vi "Laser_COM_both.vi"() -> ()   [LabVIEW 2014]
uses:
  <vilib>/Instr/_visa.llb/Select Event Type.ctl
  <vilib>/Instr/_visa.llb/VISA Configure Serial Port (Instr).vi
panel:
  in  "Freq":dbl(slide) caption="freq" min=59.9 max=1000.0 step=0.1 scale=59.9..1000.0 scale format="%#.1f"
  out "f kHz":dbl caption="Темп. модуля" format="%#_g kHz"
  out "7":bool
  out "6":bool
  out "4":bool
  out "5":bool
  out "3":bool
  out "2":bool
  out "1":bool
  out "0":bool
  out "DB25 ML":bool
  out "RS232 ML":bool
  in  "Control ML":bool
  out "on/off? 5":bool
  in  "Laser":bool
  out "Laser EM":bool caption="Излучение включено!"
  out "on/off? 3":bool
  out "on/off? 2":bool
  in  "Send":bool
  in  "write buffer":string caption="Передать команду"
  out "COM_connect":bool
  in  "Connect":bool
  out "SN:":string
  out "ID:":string
  out "Guide  laser":bool
  out "module temp":dbl caption="Темп. модуля" format="%#_g °C"
  in  "Power":dbl(slide) caption="Мощность излучения, %" min=0.0 max=100.0 step=0.5 scale=0.0..100.0 scale format="%#.2g"
  in  "Laser pilot":bool caption="Лазер пилот"
  in  "COM":refnum<visa-resource-name>="COM1" caption="Laser COM-port"
  out "read buffer":string caption="ОТВЕТ:"
  out "error out":errorcluster
  in  "error in (no error)":errorcluster
  # "ID:\n\nSN:"
  # "DB-25"
  # "RS-232"
  # "Блок  управления основным лазером"
  # "Мощьность  излучения, %"
  # "DB-25"
  # "Частота следования импульсов, кГц"
  # "T модуля -"
  # "Пилот Лазер"
  # "Терминал"
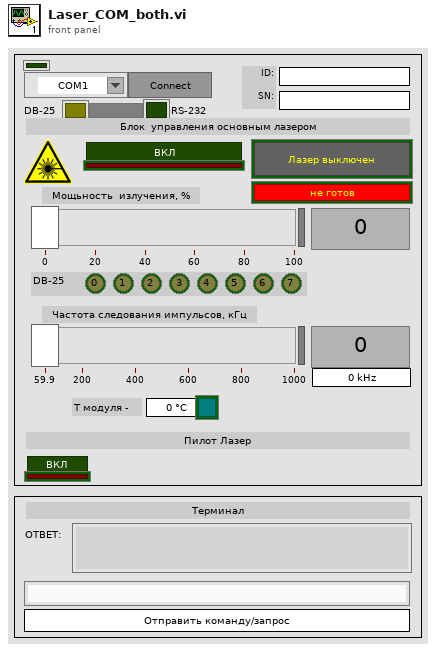
[diagram p1: front panel]
types:
  T1 = typedef "Select Event Type.ctl" = u32
  T2 = cluster{"Control by DB-25":bool, "Control by RS-232":bool, "AuxOFF control by DB-25":bool, "Guide laser control by DB-25":bool, "PRR controlled by Sync line ":bool, "Reserved[1]":bool, "The laser is in Sweep PRR mode":bool, "Modulation control by DB-25":bool, "The laser is in Jump PRR mode":bool, "Reserved[2]":bool, "Bitstream 1 (BS1) mode is active":bool, "Bitstream (BS) mode is active":bool}
  T3 = cluster{"Power control by DB-25":bool, "Reserved[1]":bool, "AuxOFF control by DB-25":bool, "Guide laser control by DB-25":bool, "Reserved[4]":bool, "Reserved[5]":bool, "Reserved[6]":bool, "Emission Modulation control by DB-25":bool, "The laser is in Jump PRR mode":bool, "Reserved[9]":bool, "Bitstream 1 (BS1) mode is active":bool, "Reserved[11]":bool, "PRR controlled by Sync line in DB-25":bool, "Emission Enable control by DB-25":bool, "APD mode is controlled by DB-25":bool, "Automatic latch":bool, "Reserved[16]":bool, "Reserved[17]":bool, "Reserved[18]":bool, "The laser is in Sweep PRR mode":bool, "The laser is in Follow PRR mode":bool, "Manual Prepump mode is active":bool, "Manual residual is controlled by DB-25":bool, "Reserved[23]":bool, "Reserved[24]":bool, "Guide laser safety function is not activated":bool, "Discharge circuit safety function is activated":bool, "Reserved[27]":bool, "Reserved[28]":bool, "Reserved[29]":bool, "Reserved[30]":bool, "Reserved[31]":bool}
  T4 = cluster{"Emergency stop":bool, "External syn frequency on pin 20 is above spec":bool, "External syn frequency on pin 20 is below spec":bool, "Laser ON time (pin 19 HIGH state) is lower spec":bool, "Laser ON time (pin 19 LOW state) is lower spec":bool, "Guide laser":bool, "Reserved [6]":bool, "Reserved [7]":bool, "Laser emission":bool, "Reserved [9]":bool, "Reserved [10]":bool, "Laser emission command was received by RS-232":bool, "Guide laser command was received by RS-232":bool, "24V Main supply voltage is in specified range":bool, "Laser uses 24V housekeeping supply":bool, "Laser uses 5V housekeeping supply":bool, "Manual Prepump is limited by it's max value 10000":bool}
  T5 = cluster{"Emergency stop":bool, "External PRR [1]":bool, "External PRR [2]":bool, "Reserved [3]":bool, "Reserved [4]":bool, "Guide laser":bool, "Reserved [6]":bool, "Reserved [7]":bool, "Laser emission":bool, "Reserved [9]":bool, "Reserved [10]":bool, "Laser emission command was received by RS-232":bool, "Guide laser command was received by RS-232":bool, "24V Main supply voltage is in specified range":bool, "HK supply voltage is in specified range":bool, "Emission Enable is switched by RS-232":bool, "Reserved [16]":bool, "Reserved [17]":bool, "Reserved [18]":bool, "Reserved [19]":bool, "Reserved [20]":bool, "Reserved [21]":bool, "Reserved [22]":bool, "Reserved [23]":bool, "Reserved [24]":bool, "Reserved [25]":bool, "Reserved [26]":bool, "Reserved [27]":bool, "Reserved [28]":bool, "Reserved [29]":bool, "Reserved [30]":bool, "Reserved [31]":bool}
  T6 = cluster{"D0 latched power setting":bool, "D1 latched power setting":bool, "D2 latched power setting":bool, "D3 latched power setting":bool, "D4 latched power setting":bool, "D5 latched power setting":bool, "D6 latched power setting":bool, "D7 latched power setting":bool, "D0 power setting":bool, "D1 power setting":bool, "D2 power setting":bool, "D3 power setting":bool, "D4 power setting":bool, "D5 power setting":bool, "D6 power setting":bool, "D7 power setting":bool, "Latch":bool, "23 AuxOFF Auxiliary Emission OFF":bool, "19 EM Emission Modulation":bool, "22 RG Guide laser control":bool, "20 Sync External Synchronization Input":bool, "18 EE Emission enable":bool, "10 Serial Input":bool, "13 Serial Clock":bool, "16 Laser status":bool, "21 Laser status":bool, "11 Laser status":bool, "12 Serial Output":bool, "24 Serial Enable":bool, "Reserved [29]":bool, "Reserved [30]":bool, "Reserved [31]":bool}
  T7 = cluster{"Module temp is out range":bool, "5V supply voltage is out range":bool, "High rack reflection":bool, "Reserved [1]":bool, "Normal Laser's status":bool, "Laser isn't ready to emmision":bool, "System error":bool, "Reserved [2]":bool}
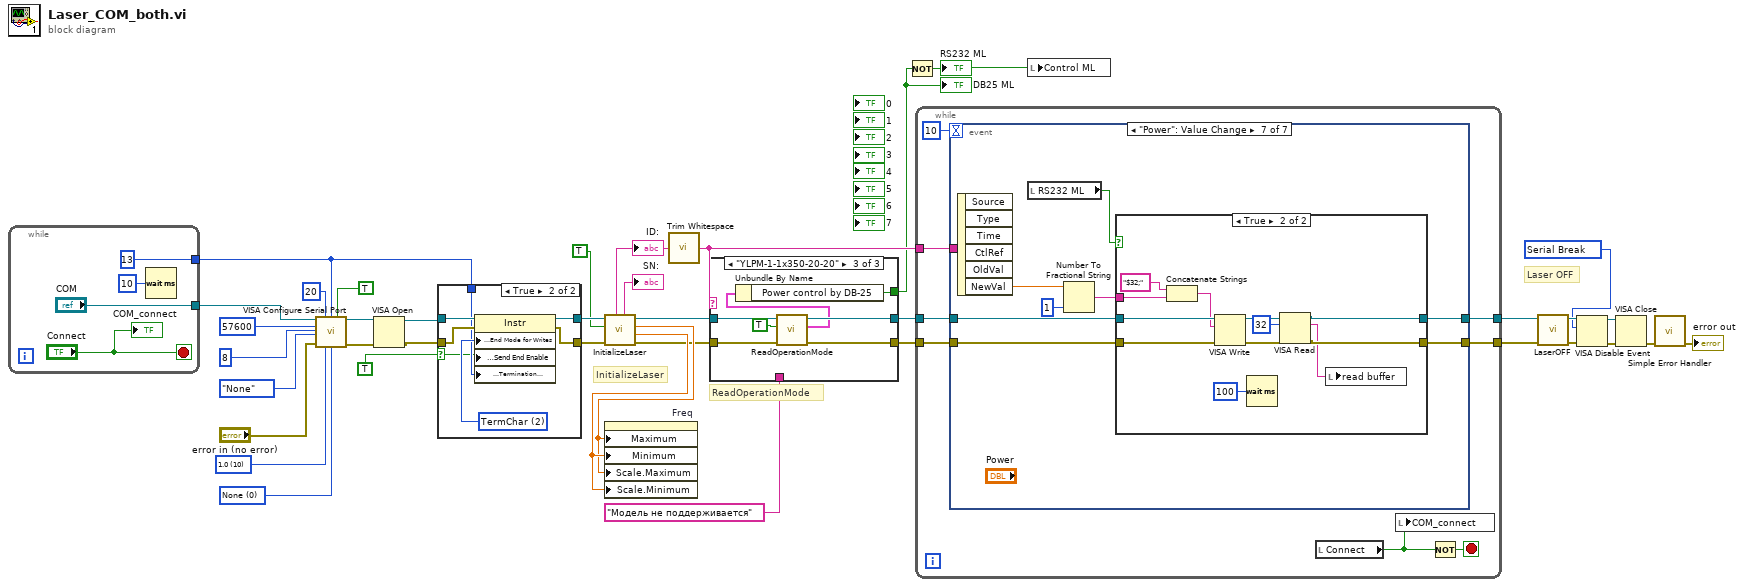
[diagram p0: block diagram]
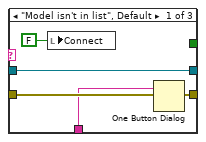
[diagram p2: hidden frame]
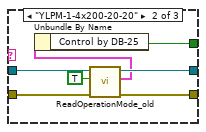
[diagram p3: hidden frame]
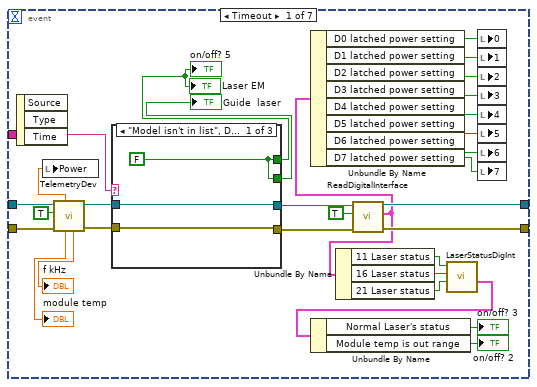
[diagram p4: hidden frame]
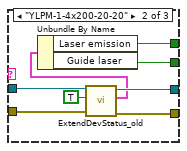
[diagram p5: hidden frame]
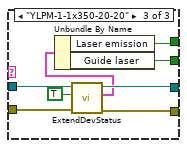
[diagram p6: hidden frame]
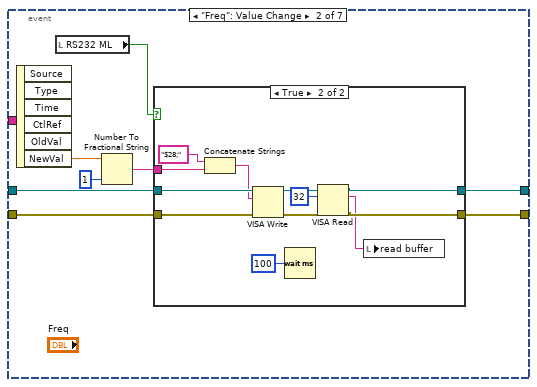
[diagram p7: hidden frame]
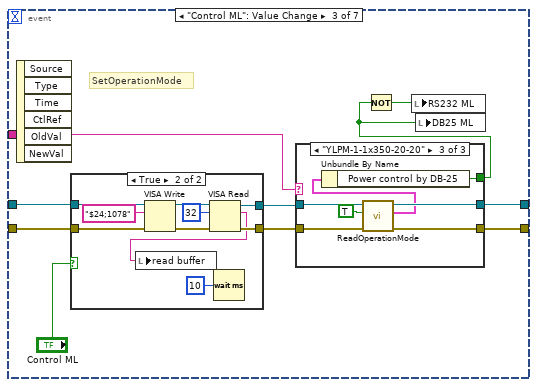
[diagram p9: hidden frame]
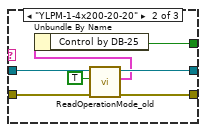
[diagram p11: hidden frame]
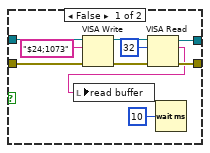
[diagram p12: hidden frame]
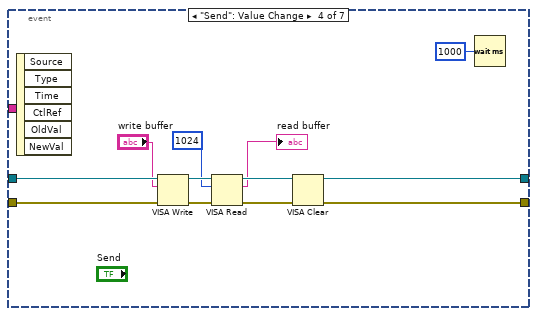
[diagram p13: hidden frame]
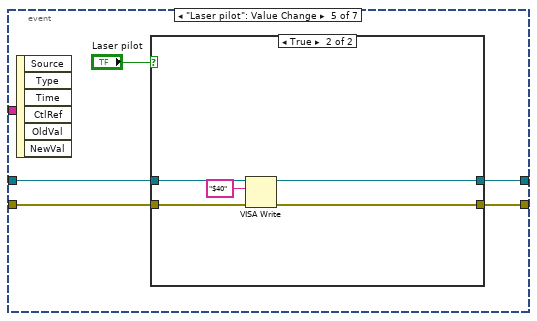
[diagram p14: hidden frame]
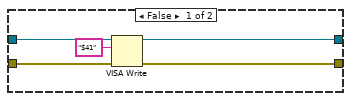
[diagram p15: hidden frame]
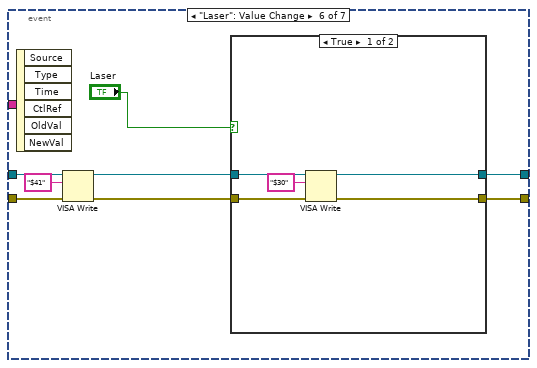
[diagram p16: hidden frame]
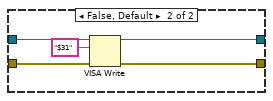
[diagram p17: hidden frame]
diagram:
  w1 = T1 1073684515 items=["Service Request"=1073684491, "Trigger"=3221168138, "Clear"=1073684493, "VXI Signal"=1073684512, "VXI/VME Interrupt"=3221168161, "VXI/VME Sysfail"=1073684509, "VXI/VME Sysreset"=1073684510, "GPIB CIC"=1073684498, "GPIB Talk"=1073684499, "GPIB Listen"=1073684500, "PXI Interrupt"=1073684514, "Serial Break"=1073684515, "Serial TermChar"=1073684516, "Serial CTS"=1073684521, "Serial DSR"=1073684522, "Serial DCD"=1073684524, "Serial RI"=1073684526, "Serial Character"=1073684533, "USB Interrupt"=1073684535, "All Enabled"=1073709055] ("Event Type")
  w25 = u16 0 items=["None", "XON/XOFF", "RTS/CTS", "XON/XOFF & RTS/CTS", "DTR/DSR", "XON/XOFF & DTR/DSR"] ("flow control (0:none)")
  w32 = u16 10 items=["1.0"=10, "1.5"=15, "2.0"=20] ("stop bits (10: 1 bit)")
  # "ReadOperationMode"
  # "Laser OFF"
  # "InitializeLaser"
  n1 = while {
    tunnel: ["COM"] -> w24
    tunnel: [i16 13 ("term_char")] -> w23
    stop <- "Connect" stop-if-true
    n2 = Wait (ms)(milliseconds to wait=u32 10) -> ()  [unwired: 1 out]
    "COM_connect" <- "Connect"
  }
  n3 = call-poly "VISA Configure Serial Port"("VISA resource name"=w24, "timeout (10sec)"=u32 20, "termination char\n(0xA = '\\n' = LF)"=w23, "Enable Termination\nChar (T)"=TRUE ("Enable Termination\nChar (T)"), "baud rate (9600)"=u32 57600 ("baud rate"), "data bits (8)"=u16 8, "parity (0:none)"=enum16{"None", "Odd", "Even", "Mark", "Space"}."None", "error in (no error)"="error in (no error)", "stop bits (10: 1 bit)"=w32, "flow control (0:none)"=w25) -> ("VISA resource name out"=w35:refnum<visa-resource-name>, "error out"=w34:errorcluster)  [unwired: 4 in]
  n4 = VISA Open(error in (no error)=w34, VISA resource name=w35) -> (VISA resource name=w29:refnum<visa-resource-name>, error out=w30:errorcluster)  [unwired: 3 in]
  n5 = case shown="True" TRUE ("End write with termination character?") {
    selector: TRUE ("End write with termination character?") -> [_ w46]
    tunnel: w29 -> [w44 w52]
    tunnel: w30 -> [w45 w51]
    tunnel: [w44 w50] -> w19
    tunnel: [w45 w49] -> w20
    tunnel: w23 -> [_ w47]
    frame False {
    }
    frame True {
      w48 = u16 2 items=["None", "LastBit", "TermChar", "Break"] ("Serial Settings:Serial End Mode for Writes")
      n6 = property class="Instr"(reference=w52, error in=w51, "Serial Settings:End Mode for Writes"=w48, "Message Based Settings:Send End Enable"=w46, "Message Based Settings:Termination Character"=w47) -> (reference out=w50:refnum<visa-resource-name>, error out=w49:errorcluster)
    }
  }
  n7 = call "InitializeLaser.vi"("error in"=w20, "ON/OFF"=TRUE, "VISA resource name in"=w19) -> ("error out"=w8:errorcluster, "Fmin"=w11:dbl, "Fmax"=w10:dbl, "VISA resource name out"=w7:refnum<visa-resource-name>, "SN:"=→"SN:":string, "Лазер: ID:"=w12:string)  [unwired: 1 in, 2 out]
  "ID:" <- w12
  n8 = property on="Freq" class="Slide (strict)"("Maximum"=w10, "Minimum"=w11, "Scale.Maximum"=w10, "Scale.Minimum"=w11) -> ()  [unwired: 2 in, 2 out]
  n9 = call <vilib>:"Trim Whitespace.vi"("string"=w12) -> ("trimmed string"=w4:string)  [unwired: 1 in]
  n10 = case shown="\"YLPM-1-1x350-20-20\"" w4 {
    tunnel: [w56 w62 w67] -> w6
    tunnel: [w54 w61 w68] -> w5
    tunnel: w7 -> [w56 w60 w70]
    tunnel: w8 -> [w54 w59 w69]
    tunnel: [_ w58 w65] -> w3
    tunnel: "Модель не поддерживается" ("error source (\" \")") -> [w53 _ _]
    frame "Model isn't in list", Default {
      n11 = local write "Connect"(FALSE ("Laser emission")) -> ()
      n12 = One Button Dialog(message=w53) -> ()  [unwired: 1 in, 1 out]
    }
    frame "YLPM-1-4x200-20-20" {
      n13 = call "ReadOperationMode_old.vi"("error in"=w59, "ON/OFF"=TRUE, "VISA resource name in"=w60) -> ("error out"=w61:errorcluster, "Operation Mode Status"=w57:T2, "VISA resource name out"=w62:refnum<visa-resource-name>)  [unwired: 5 in, 1 out]
      n14 = Unbundle By Name(w57) -> ("Control by DB-25"=w58:bool)
    }
    frame "YLPM-1-1x350-20-20" {
      n15 = call "ReadOperationMode.vi"("error in"=w69, "ON/OFF"=TRUE, "VISA resource name in"=w70) -> ("error out"=w68:errorcluster, "Operation Mode Status"=w64:T3, "VISA resource name out"=w67:refnum<visa-resource-name>)  [unwired: 5 in, 1 out]
      n16 = Unbundle By Name(w64) -> ("Power control by DB-25"=w65:bool)
    }
  }
  "DB25 ML" <- w3
  n17 = Not(x=w3) -> (.not. x?=w9:bool)
  "RS232 ML" <- w9
  n18 = while {
    tunnel: w5 -> [w73]
    tunnel: w6 -> [w74]
    tunnel: [w76] -> w17
    tunnel: [w75] -> w16
    tunnel: w4 -> [w71]
    stop <- w78 stop-if-true
    n19 = event shown="[6] \"Power\": Value Change" {
      selector: _ -> [_ _ _ _ _ _ _]
      dyn-events: _ -> [_ _ _ _ _ _ _]
      timeout: 10 -> [_ _ _ _ _ _ _]
      tunnel: w74 -> [w109 w134 w159 w208 w213 w230 w249]
      tunnel: w73 -> [w108 w133 w158 w207 w212 w229 w248]
      tunnel: [w103 w132 w156 w202 w211 w228 w245] -> w76
      tunnel: [w102 w131 w155 w201 w210 w227 w244] -> w75
      tunnel: w71 -> [w81 _ w151 _ _ _ _]
      event Timeout {
        n20 = event-data() -> ()  [unwired: 1 in, 3 out]
        n21 = call "TelemetryDev.vi"("error in"=w108, "ON/OFF"=TRUE, "VISA resource name in"=w109) -> ("error out"=w89:errorcluster, "VISA resource name out"=w90:refnum<visa-resource-name>, "Laser PRR, kHz"=→"f kHz":dbl, "module temp"=→"module temp":dbl, "Laser Power,%"=w106:dbl)  [unwired: 4 in]
        n22 = local write "Power"(w106) -> ()
        n23 = case shown="\"Model isn't in list\", Default" w81 {
          tunnel: [w112 w119 w125] -> w105
          tunnel: [w111 w118 w126] -> w104
          tunnel: w90 -> [w112 w117 w128]
          tunnel: w89 -> [w111 w116 w127]
          tunnel: [w110 w114 w121] -> w79
          tunnel: [w110 w113 w122] -> w80
          frame "Model isn't in list", Default {
            w110 = FALSE ("Laser emission")
          }
          frame "YLPM-1-4x200-20-20" {
            n24 = call "ExtendDevStatus_old.vi"("error in"=w116, "ON/OFF"=TRUE, "VISA resource name in"=w117) -> ("error out"=w118:errorcluster, "Extend Device Status"=w115:T4, "VISA resource name out"=w119:refnum<visa-resource-name>)  [unwired: 5 in]
            n25 = Unbundle By Name(w115) -> ("Laser emission"=w113:bool, "Guide laser"=w114:bool)
          }
          frame "YLPM-1-1x350-20-20" {
            n26 = call "ExtendDevStatus.vi"("error in"=w127, "ON/OFF"=TRUE, "VISA resource name in"=w128) -> ("error out"=w126:errorcluster, "Extend Device Status"=w123:T5, "VISA resource name out"=w125:refnum<visa-resource-name>)  [unwired: 5 in]
            n27 = Unbundle By Name(w123) -> ("Laser emission"=w122:bool, "Guide laser"=w121:bool)
          }
        }
        "Laser EM" <- w80
        "Guide  laser" <- w79
        "on/off? 5" <- w80
        n28 = call "ReadDigitalInterface.vi"("error in"=w104, "ON/OFF"=TRUE, "VISA resource name in"=w105) -> ("error out"=w102:errorcluster, "Extend Device Status"=w85:T6, "VISA resource name out"=w103:refnum<visa-resource-name>)  [unwired: 5 in]
        n29 = Unbundle By Name(w85) -> ("D0 latched power setting"=w91:bool, "D1 latched power setting"=w100:bool, "D2 latched power setting"=w99:bool, "D3 latched power setting"=w98:bool, "D4 latched power setting"=w97:bool, "D5 latched power setting"=w96:bool, "D6 latched power setting"=w95:bool, "D7 latched power setting"=w94:bool)
        n30 = Unbundle By Name(w85) -> ("11 Laser status"=w88:bool, "16 Laser status"=w87:bool, "21 Laser status"=w86:bool)
        n31 = call "LaserStatusDigInt.vi"("21"=w86, "16"=w87, "11"=w88) -> ("Laser Status"=w84:T7)  [unwired: 8 in]
        n32 = Unbundle By Name(w84) -> ("Normal Laser's status"=→"on/off? 3":bool, "Module temp is out range"=→"on/off? 2":bool)
        n33 = local write "0"(w91) -> ()
        n34 = local write "1"(w100) -> ()
        n35 = local write "2"(w99) -> ()
        n36 = local write "3"(w98) -> ()
        n37 = local write "4"(w97) -> ()
        n38 = local write "5"(w96) -> ()
        n39 = local write "6"(w95) -> ()
        n40 = local write "7"(w94) -> ()
      }
      event "Freq": Value Change {
        n41 = event-data() -> ("NewVal"=w129:dbl)  [unwired: 1 in, 5 out]
        n42 = local read "RS232 ML"() -> (w130:bool)
        n43 = Number To Fractional String(number=w129, precision (6)=i16 1) -> (F-format string=w136:string)  [unwired: 2 in]
        n44 = case shown="True" w130 {
          tunnel: w134 -> [w138 w150]
          tunnel: w133 -> [w137 w149]
          tunnel: w136 -> [_ w146]
          tunnel: [w138 w143] -> w132
          tunnel: [w137 w142] -> w131
          frame False {
          }
          frame True {
            n45 = Concatenate Strings("$28;" ("write buffer"), w146) -> (w147:string)
            n46 = VISA Write(VISA resource name=w150, write buffer=w147, error in (no error)=w149) -> (VISA resource name out=w145:refnum<visa-resource-name>, error out=w144:errorcluster)  [unwired: 1 out]
            n47 = Wait (ms)(milliseconds to wait=u32 100) -> ()  [unwired: 1 out]
            n48 = VISA Read(VISA resource name=w145, byte count=u32 32, error in (no error)=w144) -> (VISA resource name out=w143:refnum<visa-resource-name>, read buffer=w141:string, error out=w142:errorcluster)  [unwired: 1 out]
            n49 = local write "read buffer"(w141) -> ()
          }
        }
      }
      event "Control ML": Value Change {
        # "SetOperationMode"
        n50 = event-data() -> ()  [unwired: 1 in, 6 out]
        n51 = case shown="True" "Control ML" {
          tunnel: w159 -> [w186 w196]
          tunnel: w158 -> [w185 w195]
          tunnel: [w183 w193] -> w154
          tunnel: [w182 w192] -> w153
          frame False {
            n52 = VISA Write(VISA resource name=w186, write buffer="$24;1073", error in (no error)=w185) -> (VISA resource name out=w184:refnum<visa-resource-name>, error out=w181:errorcluster)  [unwired: 1 out]
            n53 = VISA Read(VISA resource name=w184, byte count=u32 32, error in (no error)=w181) -> (VISA resource name out=w183:refnum<visa-resource-name>, read buffer=w179:string, error out=w182:errorcluster)  [unwired: 1 out]
            n54 = local write "read buffer"(w179) -> ()
            n55 = Wait (ms)(milliseconds to wait=u32 10) -> ()  [unwired: 1 out]
          }
          frame True {
            n56 = VISA Write(VISA resource name=w196, write buffer="$24;1078", error in (no error)=w195) -> (VISA resource name out=w194:refnum<visa-resource-name>, error out=w191:errorcluster)  [unwired: 1 out]
            n57 = VISA Read(VISA resource name=w194, byte count=u32 32, error in (no error)=w191) -> (VISA resource name out=w193:refnum<visa-resource-name>, read buffer=w189:string, error out=w192:errorcluster)  [unwired: 1 out]
            n58 = local write "read buffer"(w189) -> ()
            n59 = Wait (ms)(milliseconds to wait=u32 10) -> ()  [unwired: 1 out]
          }
        }
        n60 = case shown="\"YLPM-1-1x350-20-20\"" w151 {
          tunnel: [w162 w168 w173] -> w156
          tunnel: [w161 w167 w174] -> w155
          tunnel: w154 -> [w162 w166 w176]
          tunnel: w153 -> [w161 w165 w175]
          tunnel: [_ w164 w171] -> w152
          frame "Model isn't in list", Default {
          }
          frame "YLPM-1-4x200-20-20" {
            n61 = call "ReadOperationMode_old.vi"("error in"=w165, "ON/OFF"=TRUE, "VISA resource name in"=w166) -> ("error out"=w167:errorcluster, "Operation Mode Status"=w163:T2, "VISA resource name out"=w168:refnum<visa-resource-name>)  [unwired: 5 in, 1 out]
            n62 = Unbundle By Name(w163) -> ("Control by DB-25"=w164:bool)
          }
          frame "YLPM-1-1x350-20-20" {
            n63 = call "ReadOperationMode.vi"("error in"=w175, "ON/OFF"=TRUE, "VISA resource name in"=w176) -> ("error out"=w174:errorcluster, "Operation Mode Status"=w170:T3, "VISA resource name out"=w173:refnum<visa-resource-name>)  [unwired: 5 in, 1 out]
            n64 = Unbundle By Name(w170) -> ("Power control by DB-25"=w171:bool)
          }
        }
        n65 = Not(x=w152) -> (.not. x?=w160:bool)
        n66 = local write "RS232 ML"(w160) -> ()
        n67 = local write "DB25 ML"(w152) -> ()
      }
      event "Send": Value Change {
        n68 = event-data() -> ()  [unwired: 1 in, 6 out]
        n69 = VISA Write(VISA resource name=w208, write buffer="write buffer", error in (no error)=w207) -> (VISA resource name out=w206:refnum<visa-resource-name>, error out=w205:errorcluster)  [unwired: 1 out]
        n70 = VISA Read(VISA resource name=w206, byte count=u32 1024, error in (no error)=w205) -> (VISA resource name out=w204:refnum<visa-resource-name>, read buffer=→"read buffer":string, error out=w203:errorcluster)  [unwired: 1 out]
        n71 = VISA Clear(VISA resource name=w204, error in (no error)=w203) -> (VISA resource name out=w202:refnum<visa-resource-name>, error out=w201:errorcluster)
        n72 = Wait (ms)(milliseconds to wait=u32 1000) -> ()  [unwired: 1 out]
      }
      event "Laser pilot": Value Change {
        n73 = event-data() -> ()  [unwired: 1 in, 6 out]
        n74 = case shown="True" "Laser pilot" {
          tunnel: w213 -> [w218 w223]
          tunnel: w212 -> [w217 w222]
          tunnel: [w215 w220] -> w211
          tunnel: [w214 w219] -> w210
          frame False {
            n75 = VISA Write(VISA resource name=w218, write buffer="$41", error in (no error)=w217) -> (VISA resource name out=w215:refnum<visa-resource-name>, error out=w214:errorcluster)  [unwired: 1 out]
          }
          frame True {
            n76 = VISA Write(VISA resource name=w223, write buffer="$40", error in (no error)=w222) -> (VISA resource name out=w220:refnum<visa-resource-name>, error out=w219:errorcluster)  [unwired: 1 out]
          }
        }
      }
      event "Laser": Value Change {
        n77 = event-data() -> ()  [unwired: 1 in, 6 out]
        n78 = VISA Write(VISA resource name=w230, write buffer="$41", error in (no error)=w229) -> (VISA resource name out=w226:refnum<visa-resource-name>, error out=w225:errorcluster)  [unwired: 1 out]
        n79 = case shown="True" "Laser" {
          tunnel: w226 -> [w235 w240]
          tunnel: w225 -> [w234 w239]
          tunnel: [w233 w238] -> w228
          tunnel: [w232 w237] -> w227
          frame True {
            n80 = VISA Write(VISA resource name=w235, write buffer="$30", error in (no error)=w234) -> (VISA resource name out=w233:refnum<visa-resource-name>, error out=w232:errorcluster)  [unwired: 1 out]
          }
          frame False, Default {
            n81 = VISA Write(VISA resource name=w240, write buffer="$31", error in (no error)=w239) -> (VISA resource name out=w238:refnum<visa-resource-name>, error out=w237:errorcluster)  [unwired: 1 out]
          }
        }
      }
      event "Power": Value Change {
        n82 = event-data() -> ("NewVal"=w243:dbl)  [unwired: 1 in, 5 out]
        n83 = local read "RS232 ML"() -> (w242:bool)
        n84 = Number To Fractional String(number=w243, precision (6)=i16 1) -> (F-format string=w247:string)  [unwired: 2 in]
        n85 = case shown="True" w242 {
          tunnel: w249 -> [w251 w263]
          tunnel: w248 -> [w250 w262]
          tunnel: w247 -> [_ w259]
          tunnel: [w251 w256] -> w245
          tunnel: [w250 w255] -> w244
          frame False {
          }
          frame True {
            n86 = Concatenate Strings("$32;" ("write buffer"), w259) -> (w260:string)
            n87 = VISA Write(VISA resource name=w263, write buffer=w260, error in (no error)=w262) -> (VISA resource name out=w258:refnum<visa-resource-name>, error out=w257:errorcluster)  [unwired: 1 out]
            n88 = Wait (ms)(milliseconds to wait=u32 100) -> ()  [unwired: 1 out]
            n89 = VISA Read(VISA resource name=w258, byte count=u32 32, error in (no error)=w257) -> (VISA resource name out=w256:refnum<visa-resource-name>, read buffer=w254:string, error out=w255:errorcluster)  [unwired: 1 out]
            n90 = local write "read buffer"(w254) -> ()
          }
        }
      }
    }
    n91 = local read "Connect"() -> (w77:bool)
    n92 = local write "COM_connect"(w77) -> ()
    n93 = Not(x=w77) -> (.not. x?=w78:bool)
  }
  n94 = local write "Control ML"(w9) -> ()
  n95 = call "LaserOFF.vi"("error in"=w16, "VISA resource name in"=w17) -> ("error out"=w13:errorcluster, "VISA resource name out"=w14:refnum<visa-resource-name>)  [unwired: 8 in]
  n96 = VISA Disable Event(8:w13, 10:w1, 11:w14) -> (0:w21:errorcluster, 3:w22:refnum<visa-resource-name>)  [unwired: 1 out]
  n97 = VISA Close(VISA resource name=w22, error in (no error)=w21) -> (error out=w26:errorcluster)
  n98 = call <vilib>:"Simple Error Handler.vi"("error in (no error)"=w26) -> ("error out"=→"error out":errorcluster)  [unwired: 4 in, 4 out]
